vi "XY Graph Set Cursor Style.vi"(6 "Cursor Color (Panel & Object Text)":u32(colorbox)=16777222, 8 "Error In":errorcluster, 9 "Cursor Style (Crosshair)":u8=8, 10 "Point Style (Open Circle)":u8=1, 11 "XYGraph Refnum":refnum<vi>) -> (0 "Error Out":errorcluster, 3 "XYGraph Refnum (dup)":refnum<vi>)   [LabVIEW 2021, in "XY Graph Add-Ons.lvlib"]
uses:
  XY Graph Add-Ons.lvlib
  Arrays/Arrays.lvlib
panel:
  in  "Cursor index (-1: last)":i32
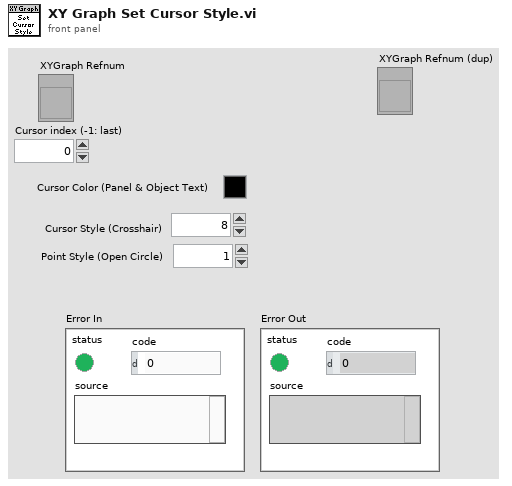
[diagram p1: front panel]
types:
  T1 = typedef "LVCursorListTypeDef.ctl" = cluster{"Name":string, "Color":u32, "Style":u8, "Point Style":u8, "Name Visible":bool, "Allow Drag":bool, "Cursor Mode":u32, "Plot":i32, "Index":i32, "Position":cluster{"X":dbl, "Y":dbl}, "X Scale":u32, "Y Scale":u32, "Watch Plots":i32[], "Watch All Plots":bool, "Plot Area":i32, "Label Offset":cluster{"X":dbl, "Y":dbl}}[]
  T2 = cluster{"Name":string, "Color":u32, "Style":u8, "Point Style":u8, "Name Visible":bool, "Allow Drag":bool, "Cursor Mode":u32, "Plot":i32, "Index":i32, "Position":cluster{"X":dbl, "Y":dbl}, "X Scale":u32, "Y Scale":u32, "Watch Plots":i32[], "Watch All Plots":bool, "Plot Area":i32, "Label Offset":cluster{"X":dbl, "Y":dbl}}
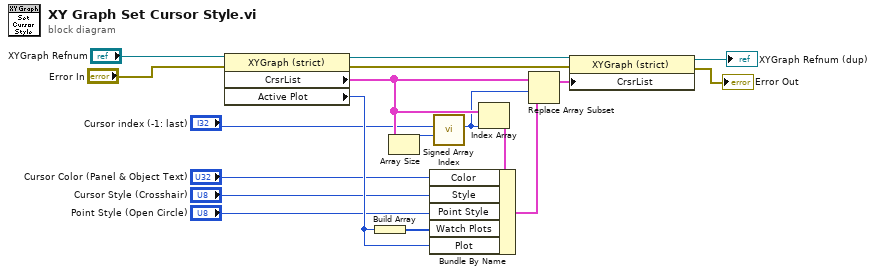
[diagram p0: block diagram]
diagram:
  n1 = property class="XYGraph (strict)"(reference="XYGraph Refnum", error in="Error In") -> (reference out=w13:refnum<vi>, error out=w1:errorcluster, "CrsrList"=w9:T1, "Active Plot"=w18:u32)
  n2 = Build Array(w18) -> (w14:u32[])
  n3 = Array Size(array=w9) -> (size(s)=w8:i32)
  n4 = call "Signed Array Index.vi"("Array Size"=w8, "Array Index in"="Cursor index (-1: last)") -> ("Array Index out"=w5:i32)  [unwired: 9 in]
  n5 = Index Array(array=w9, index=w5) -> (element=w6:T2)
  n6 = Bundle By Name(cluster=w6, "Color"="Cursor Color (Panel & Object Text)", "Style"="Cursor Style (Crosshair)", "Point Style"="Point Style (Open Circle)", "Watch Plots"=w14, "Plot"=w18) -> (w4:T2)
  n7 = Replace Array Subset(array=w9, new element=w4, index=w5) -> (w10:T1)
  n8 = property class="XYGraph (strict)"(reference=w13, error in=w1, "CrsrList"=w10) -> (reference out=→"XYGraph Refnum (dup)":refnum<vi>, error out=→"Error Out":errorcluster)
